vi "Teleop.vi"(10 "Match Info":T1={"Autonomous Elapsed Seconds"=0.0, "TeleOp Elapsed Seconds"=0.0, "Disabled Elapsed Seconds"=0.0, "Visited Autonomous"=FALSE, "Visited TeleOp"=FALSE, "Visited Disabled"=FALSE, "Autonomous Settings"={"Autonomous Style"=enum."Independent", "VI Refnum"=refnum}}, 11 "Call Context":T2) -> ()   [LabVIEW 2013]
doc: "This VI is called for each TeleOp packet received from the DS where the robot is not disabled. It is often used to read from the joysticks and update I/O or to update setpoints for timed control loops. It should complete and return within 20 milliseconds or it may miss DS packets."
uses:
  Robot Global Data.vi
  <vilib>/Rock Robotics/WPI/DriverStation/WPI_DriverStationMatch Info.ctl
  <vilib>/Rock Robotics/WPI/DriverStation/WPI_DriverStationDerivedRobotMode.ctl
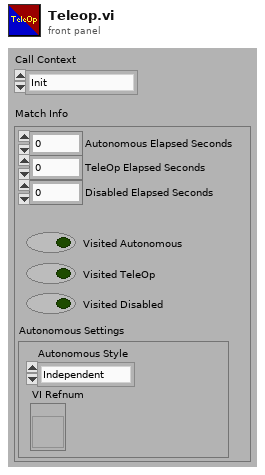
[diagram p1: front panel]
types:
  T1 = typedef "WPI_DriverStationMatch Info.ctl" = cluster{"Autonomous Elapsed Seconds":dbl, "TeleOp Elapsed Seconds":dbl, "Disabled Elapsed Seconds":dbl, "Visited Autonomous":bool, "Visited TeleOp":bool, "Visited Disabled":bool, "Autonomous Settings":cluster{"Autonomous Style":enum16{"Iterative", "Independent"}, "VI Refnum":refnum<vi>}}
  T2 = typedef "WPI_DriverStationDerivedRobotMode.ctl" = enum16{"Init", "Execute", "Stop"}
  T3 = typedef "WPI_JoystickDevRef.ctl" = cluster{"Device":T4}
  T4 = typedef "WPI_JoystickDeviceEnum.ctl" = enum16{"USB 1", "USB 2", "USB 3", "USB 4", "Kinect 1", "Kinect 2"}
  T5 = typedef "WPI_GyroDevRef.ctl" = cluster{"DevStatus":errorcluster, "Analog Module":T6, "Analog Channel":T7, "Offset":dbl, "Gain (VoltsPerDegree/Second)":dbl}
  T6 = typedef "FPGA_TypedefAnalogModule.ctl" = enum16{"Analog Module 1", "Analog Module 2"}
  T7 = typedef "FPGA_AIChannel.ctl" = enum8{"AI 1", "AI 2", "AI 3", "AI 4", "AI 5", "AI 6", "AI 7", "AI 8", "Invalid"}
  T8 = typedef "WPI_JoystickButtonState.ctl" = cluster{"Button 1":bool, "Button 2":bool, "Button 3":bool, "Button 4":bool, "Button 5":bool, "Button 6":bool, "Button 7":bool, "Button 8":bool, "Button 9":bool, "Button 10":bool, "Button 11":bool, "Button 12":bool}
  T9 = cluster{"axis 1 (x)":dbl, "axis 2 (y)":dbl, "axis 3 (throttle)":dbl, "axis 4":dbl, "axis 5":dbl, "axis 6":dbl}
  T10 = typedef "WPI_AnalogChannelDevRef.ctl" = cluster{"DevStatus":errorcluster, "Analog Module":T6, "Analog Channel":T7}
  T11 = typedef "WPI_DigitalInputDevRef.ctl" = cluster{"DevStatus":errorcluster, "DIO Channel":T12, "Digital Module":T13}
  T12 = typedef "FPGA_DIOChannel.ctl" = enum8{"DIO 1", "DIO 2", "DIO 3", "DIO 4", "DIO 5", "DIO 6", "DIO 7", "DIO 8", "DIO 9", "DIO 10", "DIO 11", "DIO 12", "DIO 13", "DIO 14", "Invalid"}
  T13 = typedef "FPGA_TypedefDigitalModule.ctl" = enum16{"Digital Module 1", "Digital Module 2"}
  T14 = typedef "WPI_RobotDriveDevRef.ctl" = cluster{"DevStatus":errorcluster, "Motors[]":T15[], "Square Inputs":bool, "Max Output":dbl, "Isochronous":bool}
  T15 = typedef "WPI_MotorControlDeviceRef.ctl" = cluster{"DeviceStatus":errorcluster, "Type":enum16{"PWM", "CAN"}, "PWM":cluster{"Digital Module":T13, "PWM Channel":T16, "DeadBand":T17}, "CAN":cluster{"Device Number":u8, "Control Mode":T18, "Semaphore":T19, "Max Vout":dbl}, "Invert":bool, "TransformRef":T20, "InvTransformRef":T20}
  T16 = typedef "FPGA_DIOPWMChannel.ctl" = enum8{"PWM 1", "PWM 2", "PWM 3", "PWM 4", "PWM 5", "PWM 6", "PWM 7", "PWM 8", "PWM 9", "PWM 10", "Invalid"}
  T17 = typedef "WPI_PWMDeadband.ctl" = cluster{"Name":string, "maxPositivePwm":i32, "minPositivePwm":i32, "centerPwm":i32, "maxNegativePwm":i32, "minNegativePwm":i32, "angularRange":u16}
  T18 = typedef "WPI_CANJaguar_ControlMode.ctl" = enum8{"Percent VBus", "Current", "Speed", "Position", "Voltage"}
  T19 = typedef "Semaphore RefNum" = refnum<k1>
  T20 = typedef "WPI_PWMTransform_ConPane.ctl" = refnum<vi>
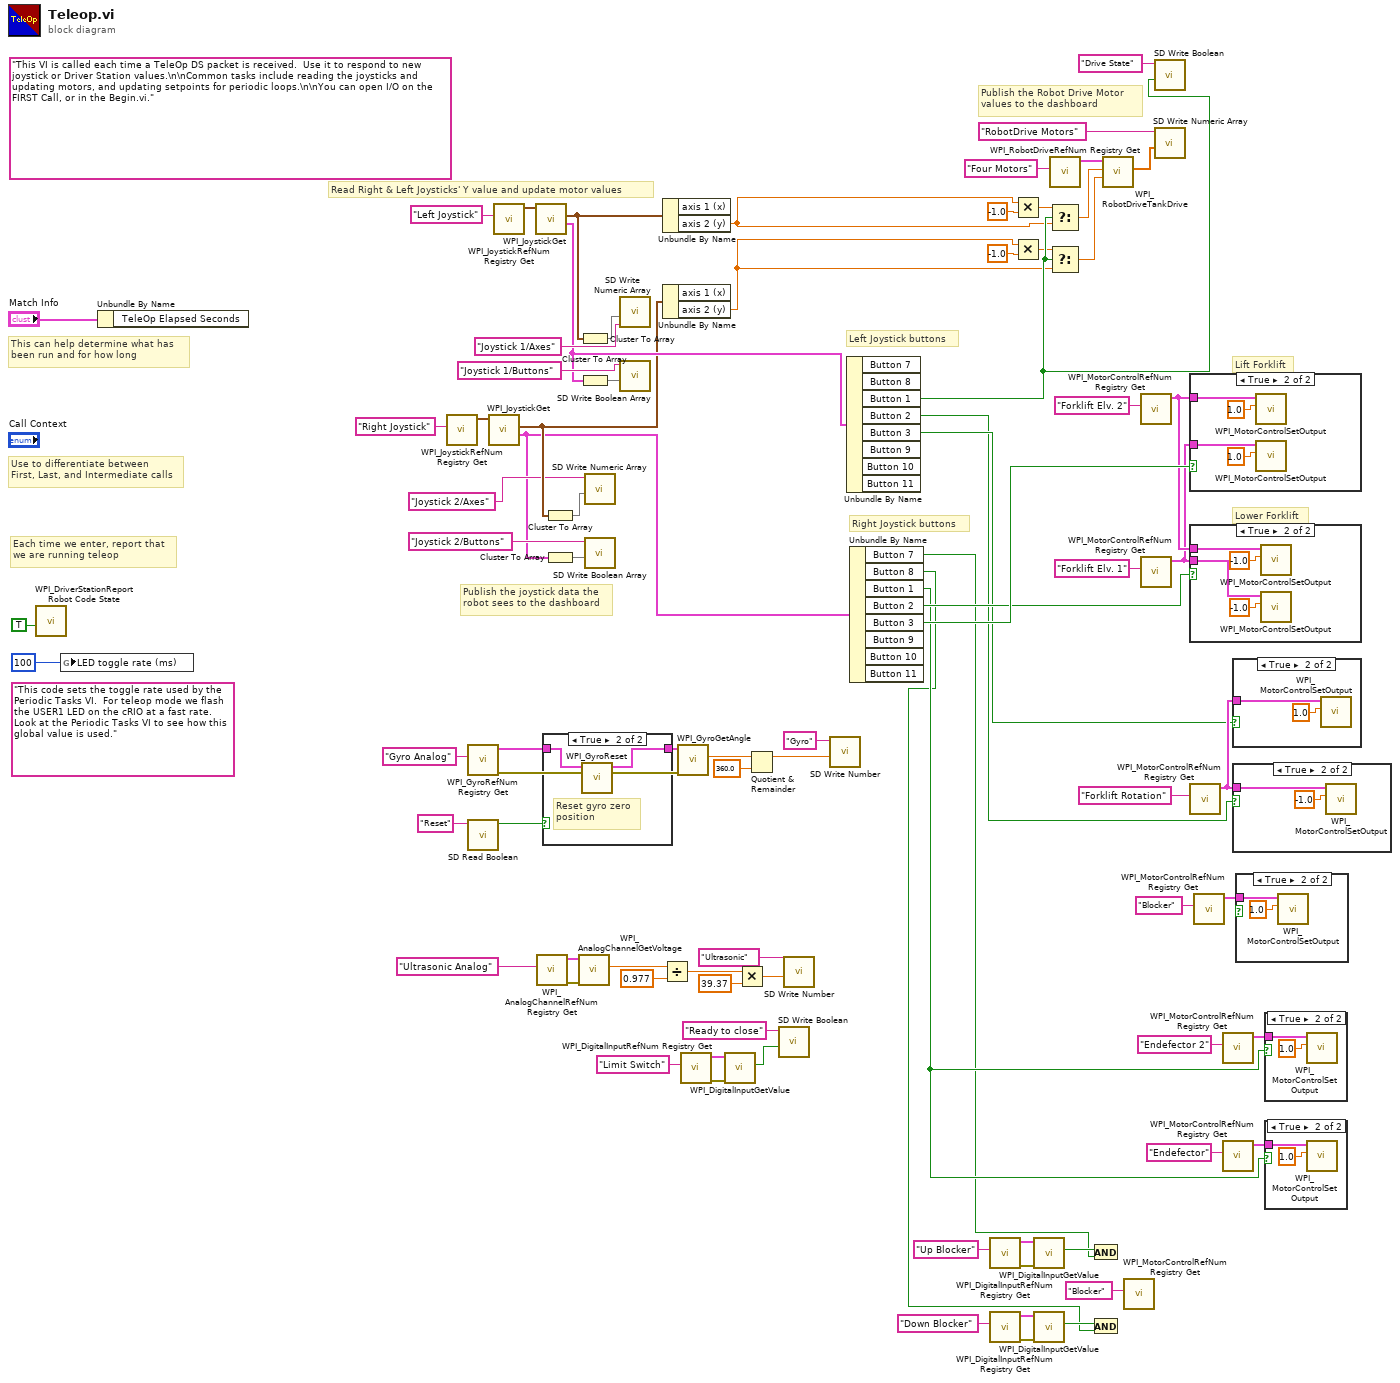
[diagram p0: block diagram]
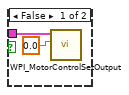
[diagram p3: hidden frame]
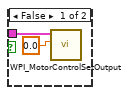
[diagram p4: hidden frame]
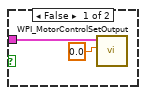
[diagram p5: hidden frame]
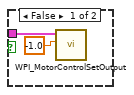
[diagram p6: hidden frame]
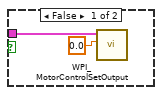
[diagram p7: hidden frame]
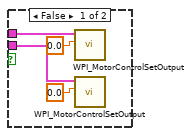
[diagram p8: hidden frame]
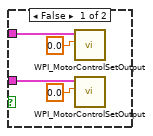
[diagram p9: hidden frame]
diagram:
  (unwired) "This code sets the toggle rate used by the Periodic Tasks VI.  For teleop mode we flash the USER1 LED on the cRIO at a fast rate.  Look at the Periodic Tasks VI to see how this global value is used."
  (unwired) "This VI is called each time a TeleOp DS packet is received.  Use it to respond to new joystick or Driver Station values.\n\nCommon tasks include reading the joysticks and updating motors, and updating setpoints for periodic loops.\n\nYou can open I/O on the FIRST Call, or in the Begin.vi."
  # "Publish the joystick data the\nrobot sees to the dashboard"
  # "Right Joystick buttons"
  # "Left Joystick buttons"
  # "Lower Forklift"
  # "Lift Forklift"
  # "Publish the Robot Drive Motor\nvalues to the dashboard"
  # "Read Right & Left Joysticks' Y value and update motor values"
  # "Each time we enter, report that\nwe are running teleop"
  # "Use to differentiate between\nFirst, Last, and Intermediate calls"
  # "This can help determine what has\nbeen run and for how long"
  n1 = call <vilib>:"WPI_DriverStationReport Robot Code State.vi"("TeleOp"=TRUE ("Autonomous")) -> ()  [unwired: 10 in, 1 out]
  n2 = global write "Robot Global Data.vi" "LED toggle rate (ms)"(u32 100 ("LED ms toggle rate")) -> ()
  n3 = Unbundle By Name("Match Info") -> ()  [unwired: 1 out]
  n4 = call <vilib>:"WPI_JoystickRefNum Registry Get.vi"("refnum name"="Right Joystick") -> ("JoystickDevRef"=w72:T3)  [unwired: 1 in, 9 out]
  n5 = call <vilib>:"WPI_GyroRefNum Registry Get.vi"("refnum name"="Gyro Analog") -> ("error out"=w35:errorcluster, "GyroDevRef"=w29:T5)  [unwired: 9 in]
  n6 = call <vilib>:"SD Read Boolean.vi"("Name"="Reset") -> ("Boolean"=w27:bool)  [unwired: 8 in, 2 out]
  n7 = call <vilib>:"WPI_JoystickGet.vi"("JoystickDevRef"=w72) -> ("Buttons"=w66:T8, "Axes"=w69:T9)  [unwired: 1 in, 4 out]
  n8 = call <vilib>:"WPI_JoystickRefNum Registry Get.vi"("refnum name"="Left Joystick") -> ("JoystickDevRef"=w81:T3)  [unwired: 1 in, 9 out]
  n9 = call <vilib>:"WPI_JoystickGet.vi"("JoystickDevRef"=w81) -> ("Buttons"=w74:T8, "Axes"=w78:T9)  [unwired: 1 in, 4 out]
  n10 = call <vilib>:"WPI_AnalogChannelRefNum Registry Get.vi"("refnum name"="Ultrasonic Analog") -> ("error out"=w17:errorcluster, "AIDeviceRef"=w19:T10)  [unwired: 9 in]
  n11 = case shown="True" w27 {
    tunnel: w29 -> [w86 w88]
    tunnel: [w86 w87] -> w28
    frame False {
    }
    frame True {
      # "Reset gyro zero \nposition"
      n12 = call <vilib>:"WPI_GyroReset.vi"("GyroDevRef"=w88) -> ("GyroDevRef"=w87:T5)  [unwired: 10 out]
    }
  }
  n13 = Cluster To Array(cluster=w69) -> (array=w68:dbl[])
  n14 = Cluster To Array(cluster=w66) -> (array=w71:bool[])
  n15 = call <vilib>:"WPI_AnalogChannelGetVoltage.vi"("error in (no error)"=w17, "AIDeviceRef"=w19) -> ("Voltage"=w20:dbl)  [unwired: 7 in, 2 out]
  n16 = Cluster To Array(cluster=w78) -> (array=w77:dbl[])
  n17 = Cluster To Array(cluster=w74) -> (array=w80:bool[])
  n18 = call <vilib>:"SD Write Numeric Array.vi"("Numeric Array"=w68, "Name"="Joystick 2/Axes") -> ()  [unwired: 8 in, 2 out]
  n19 = call <vilib>:"SD Write Boolean Array.vi"("Boolean Array"=w71, "Name"="Joystick 2/Buttons") -> ()  [unwired: 8 in, 2 out]
  n20 = call <vilib>:"SD Write Numeric Array.vi"("Numeric Array"=w77, "Name"="Joystick 1/Axes") -> ()  [unwired: 8 in, 2 out]
  n21 = call <vilib>:"SD Write Boolean Array.vi"("Boolean Array"=w80, "Name"="Joystick 1/Buttons") -> ()  [unwired: 8 in, 2 out]
  n22 = Divide(x=w20, y=0.977 ("Output")) -> (x/y=w23:dbl)
  n23 = Unbundle By Name(w78) -> ("axis 2 (y)"=w38:dbl)  [unwired: 1 out]
  n24 = Unbundle By Name(w69) -> ("axis 2 (y)"=w37:dbl)  [unwired: 1 out]
  n25 = call <vilib>:"WPI_GyroGetAngle.vi"("error in (no error)"=w35, "GyroDevRef"=w28) -> ("Angle"=w33:dbl)  [unwired: 6 in, 3 out]
  n26 = call <vilib>:"WPI_DigitalInputRefNum Registry Get.vi"("refnum name"="Limit Switch") -> ("error out"=w16:errorcluster, "DigitalInputDevRef"=w15:T11)  [unwired: 9 in]
  n27 = call <vilib>:"WPI_DigitalInputGetValue.vi"("error in (no error)"=w16, "DigitalInputDevRef"=w15) -> ("Value"=w13:bool)  [unwired: 7 in, 2 out]
  n28 = Multiply(x=w23, y=39.37 ("Output")) -> (x*y=w25:dbl)
  n29 = Quotient & Remainder(x=w33, y=360.0) -> (x-y*floor(x/y)=w31:dbl)  [unwired: 1 out]
  n30 = call <vilib>:"SD Write Boolean.vi"("Boolean"=w13, "Name"="Ready to close") -> ()  [unwired: 8 in, 2 out]
  n31 = call <vilib>:"SD Write Number.vi"("Numeric"=w25, "Name"="Ultrasonic") -> ()  [unwired: 8 in, 2 out]
  n32 = call <vilib>:"SD Write Number.vi"("Numeric"=w31, "Name"="Gyro") -> ()  [unwired: 8 in, 2 out]
  n33 = Unbundle By Name(w74) -> ("Button 1"=w44:bool, "Button 2"=w36:bool, "Button 3"=w54:bool)  [unwired: 5 out]
  n34 = Unbundle By Name(w66) -> ("Button 7"=w3:bool, "Button 8"=w2:bool, "Button 1"=w48:bool, "Button 2"=w56:bool, "Button 3"=w64:bool)  [unwired: 3 out]
  n35 = call <vilib>:"WPI_DigitalInputRefNum Registry Get.vi"("refnum name"="Up Blocker") -> ("error out"=w11:errorcluster, "DigitalInputDevRef"=w10:T11)  [unwired: 9 in]
  n36 = call <vilib>:"WPI_DigitalInputRefNum Registry Get.vi"("refnum name"="Down Blocker") -> ("error out"=w7:errorcluster, "DigitalInputDevRef"=w6:T11)  [unwired: 9 in]
  n37 = Multiply(x=w38, y=-1.0) -> (x*y=w43:dbl)
  n38 = Multiply(x=w37, y=-1.0) -> (x*y=w40:dbl)
  n39 = call <vilib>:"WPI_DigitalInputGetValue.vi"("error in (no error)"=w11, "DigitalInputDevRef"=w10) -> ("Value"=w8:bool)  [unwired: 7 in, 2 out]
  n40 = call <vilib>:"WPI_DigitalInputGetValue.vi"("error in (no error)"=w7, "DigitalInputDevRef"=w6) -> ("Value"=w4:bool)  [unwired: 7 in, 2 out]
  n41 = call <vilib>:"WPI_RobotDriveRefNum Registry Get.vi"("refnum name"="Four Motors") -> ("RobotDriveDevRef"=w39:T14)  [unwired: 1 in, 9 out]
  n42 = Select(t=w43, s=w44, f=w38) -> (s? t:f=w47:dbl)
  n43 = Select(t=w40, s=w44, f=w37) -> (s? t:f=w46:dbl)
  n44 = And(x=w8, y=w3) -> ()  [unwired: 1 out]
  n45 = And(x=w4, y=w2) -> ()  [unwired: 1 out]
  n46 = call <vilib>:"WPI_RobotDriveTankDrive.vi"("Right axis value"=w46, "Left axis value"=w47, "RobotDriveDevRef"=w39) -> ("Motor Values"=w45:dbl[])  [unwired: 6 in, 2 out]
  n47 = call <vilib>:"WPI_MotorControlRefNum Registry Get.vi"("refnum name"="Blocker") -> ()  [unwired: 9 in, 2 out]
  n48 = call <vilib>:"WPI_MotorControlRefNum Registry Get.vi"("refnum name"="Forklift Elv. 2") -> ("MotorControlDevRef"=w61:T15)  [unwired: 9 in, 1 out]
  n49 = call <vilib>:"WPI_MotorControlRefNum Registry Get.vi"("refnum name"="Forklift Elv. 1") -> ("MotorControlDevRef"=w60:T15)  [unwired: 9 in, 1 out]
  n50 = call <vilib>:"SD Write Boolean.vi"("Boolean"=w44, "Name"="Drive State") -> ()  [unwired: 8 in, 2 out]
  n51 = call <vilib>:"SD Write Numeric Array.vi"("Numeric Array"=w45, "Name"="RobotDrive Motors") -> ()  [unwired: 8 in, 2 out]
  n52 = case shown="True" w64 {
    tunnel: w61 -> [w89 w95]
    tunnel: w60 -> [w90 w96]
    frame False {
      n53 = call <vilib>:"WPI_MotorControlSetOutput.vi"("Output"=0.0, "MotorControlDevRef"=w89) -> ()  [unwired: 7 in, 3 out]
      n54 = call <vilib>:"WPI_MotorControlSetOutput.vi"("Output"=0.0, "MotorControlDevRef"=w90) -> ()  [unwired: 7 in, 3 out]
    }
    frame True {
      n55 = call <vilib>:"WPI_MotorControlSetOutput.vi"("Output"=1.0, "MotorControlDevRef"=w95) -> ()  [unwired: 7 in, 3 out]
      n56 = call <vilib>:"WPI_MotorControlSetOutput.vi"("Output"=1.0, "MotorControlDevRef"=w96) -> ()  [unwired: 7 in, 3 out]
    }
  }
  n57 = case shown="True" w56 {
    tunnel: w61 -> [w97 w103]
    tunnel: w60 -> [w98 w104]
    frame False {
      n58 = call <vilib>:"WPI_MotorControlSetOutput.vi"("Output"=0.0, "MotorControlDevRef"=w97) -> ()  [unwired: 7 in, 3 out]
      n59 = call <vilib>:"WPI_MotorControlSetOutput.vi"("Output"=0.0, "MotorControlDevRef"=w98) -> ()  [unwired: 7 in, 3 out]
    }
    frame True {
      n60 = call <vilib>:"WPI_MotorControlSetOutput.vi"("Output"=-1.0, "MotorControlDevRef"=w103) -> ()  [unwired: 7 in, 3 out]
      n61 = call <vilib>:"WPI_MotorControlSetOutput.vi"("Output"=-1.0, "MotorControlDevRef"=w104) -> ()  [unwired: 7 in, 3 out]
    }
  }
  n62 = call <vilib>:"WPI_MotorControlRefNum Registry Get.vi"("refnum name"="Forklift Rotation") -> ("MotorControlDevRef"=w55:T15)  [unwired: 9 in, 1 out]
  n63 = call <vilib>:"WPI_MotorControlRefNum Registry Get.vi"("refnum name"="Blocker") -> ("MotorControlDevRef"=w57:T15)  [unwired: 9 in, 1 out]
  n64 = call <vilib>:"WPI_MotorControlRefNum Registry Get.vi"("refnum name"="Endefector 2") -> ("MotorControlDevRef"=w49:T15)  [unwired: 9 in, 1 out]
  n65 = call <vilib>:"WPI_MotorControlRefNum Registry Get.vi"("refnum name"="Endefector") -> ("MotorControlDevRef"=w50:T15)  [unwired: 9 in, 1 out]
  n66 = case shown="True" w54 {
    tunnel: w55 -> [w105 w107]
    frame False {
      n67 = call <vilib>:"WPI_MotorControlSetOutput.vi"("Output"=0.0, "MotorControlDevRef"=w105) -> ()  [unwired: 7 in, 3 out]
    }
    frame True {
      n68 = call <vilib>:"WPI_MotorControlSetOutput.vi"("Output"=1.0, "MotorControlDevRef"=w107) -> ()  [unwired: 7 in, 3 out]
    }
  }
  n69 = case shown="True" w36 {
    tunnel: w55 -> [w109 w111]
    frame False {
      n70 = call <vilib>:"WPI_MotorControlSetOutput.vi"("Output"=0.0, "MotorControlDevRef"=w109) -> ()  [unwired: 7 in, 3 out]
    }
    frame True {
      n71 = call <vilib>:"WPI_MotorControlSetOutput.vi"("Output"=-1.0, "MotorControlDevRef"=w111) -> ()  [unwired: 7 in, 3 out]
    }
  }
  n72 = case shown="True" {
    selector: _ -> [_ _]
    tunnel: w57 -> [w113 w115]
    frame False {
      n73 = call <vilib>:"WPI_MotorControlSetOutput.vi"("Output"=-1.0, "MotorControlDevRef"=w113) -> ()  [unwired: 7 in, 3 out]
    }
    frame True {
      n74 = call <vilib>:"WPI_MotorControlSetOutput.vi"("Output"=1.0, "MotorControlDevRef"=w115) -> ()  [unwired: 7 in, 3 out]
    }
  }
  n75 = case shown="True" w48 {
    tunnel: w49 -> [w117 w119]
    frame False {
      n76 = call <vilib>:"WPI_MotorControlSetOutput.vi"("Output"=0.0, "MotorControlDevRef"=w117) -> ()  [unwired: 7 in, 3 out]
    }
    frame True {
      n77 = call <vilib>:"WPI_MotorControlSetOutput.vi"("Output"=1.0, "MotorControlDevRef"=w119) -> ()  [unwired: 7 in, 3 out]
    }
  }
  n78 = case shown="True" w48 {
    tunnel: w50 -> [w121 w123]
    frame False {
      n79 = call <vilib>:"WPI_MotorControlSetOutput.vi"("Output"=0.0, "MotorControlDevRef"=w121) -> ()  [unwired: 7 in, 3 out]
    }
    frame True {
      n80 = call <vilib>:"WPI_MotorControlSetOutput.vi"("Output"=1.0, "MotorControlDevRef"=w123) -> ()  [unwired: 7 in, 3 out]
    }
  }
